vi "LuminosidadyTemperatura.vi"() -> ()   [LabVIEW 2021]
panel:
  out "Luz3":bool
  out "Luz2":bool
  in  "Sensor Presencia 3":bool
  in  "Sensor Presencia 2":bool
  in  "Sensor fotoelectrico":bool
  in  "Sensor Presencia 1":bool
  out "Calefactor":bool
  out "Ventilador":bool
  out "Indicador Analogico":dbl(knob) scale=0.0..45.0
  out "IndicadorTemp":dbl
  in  "Temperatura":dbl=15.0 min=15.0 max=26.0
  in  "ControlLuminosidad":dbl
  out "Luz1":bool
  out "Indicador 2":dbl
  out "Indicador":dbl
  out "Iluminacion 3":dbl(slide) scale=0.0..100.0
  out "Iluminacion 2":dbl(slide) scale=0.0..100.0
  out "Iluminacion 1":dbl(slide) scale=0.0..100.0
  out "Datos para DAQ 1":dbl
  in  "stop":bool
  # "Tablero de Monitoreo"
  # "Control de Luminosidad"
  # "Control de Temperatura"
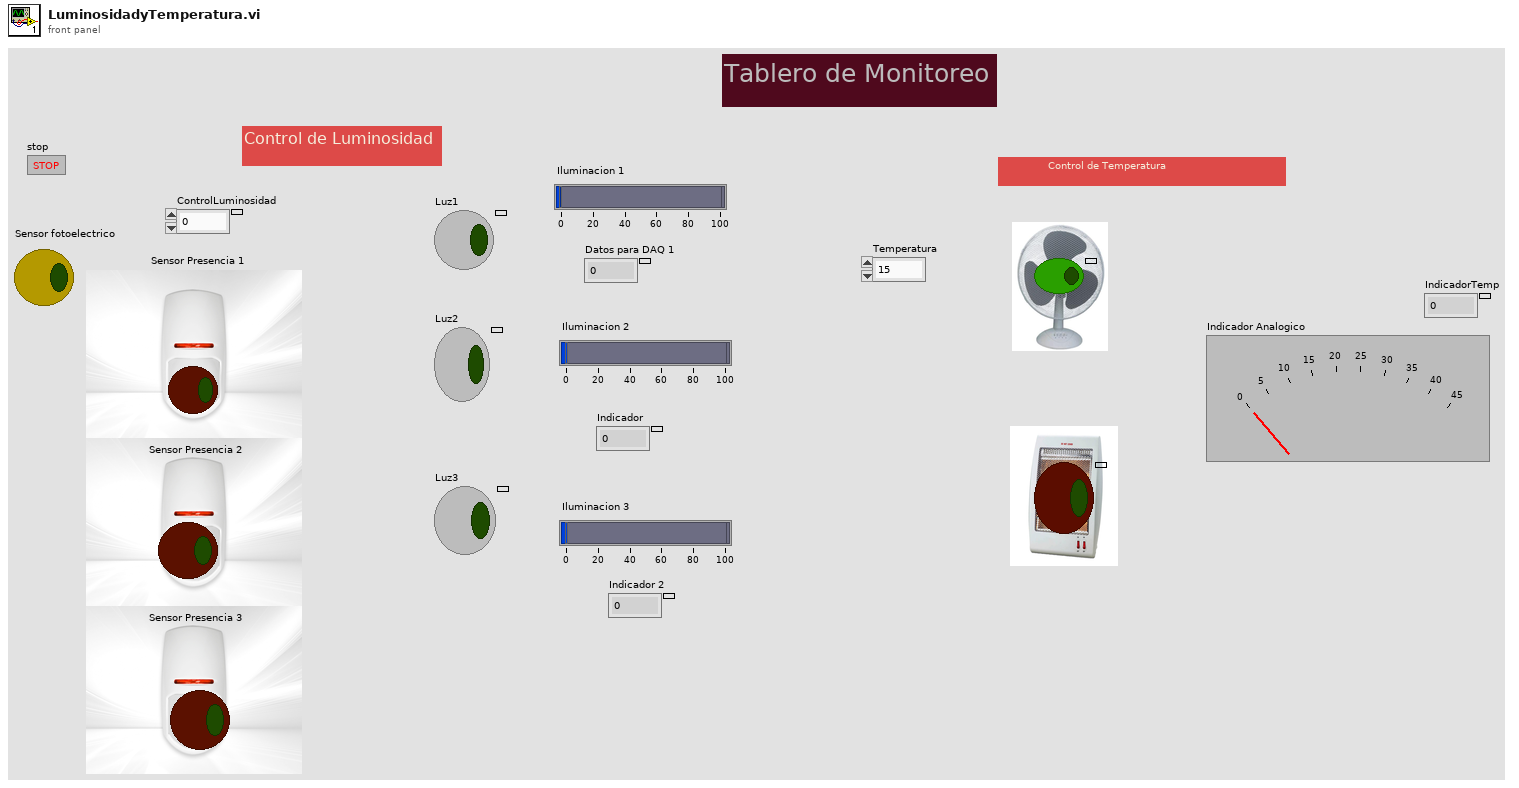
[diagram p1: front panel]
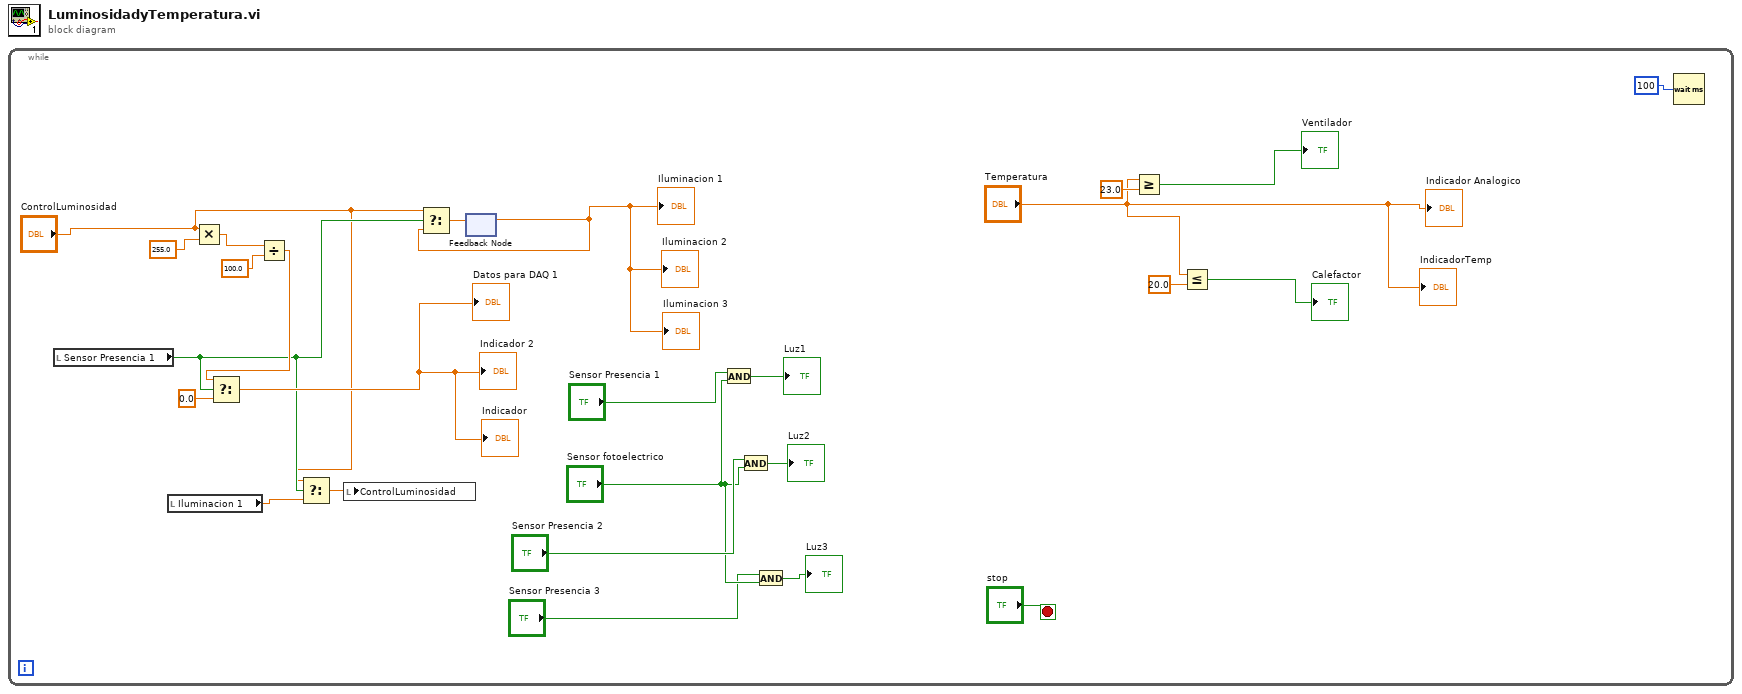
[diagram p0: block diagram]
diagram:
  n1 = while {
    stop <- "stop" stop-if-true
    n2 = local read "Sensor Presencia 1"() -> (w16:bool)
    n3 = local read "Iluminacion 1"() -> (w15:dbl)
    n4 = Multiply(x="ControlLuminosidad", y=255.0) -> (x*y=w23:dbl)
    n5 = Divide(x=w23, y=100.0) -> (x/y=w21:dbl)
    n6 = Select(t=w21, s=w16, f=0.0) -> (s? t:f=→"Datos para DAQ 1" →"Indicador 2" →"Indicador":dbl)
    n7 = Select(t="ControlLuminosidad", s=w16, f=w15) -> (s? t:f=w14:dbl)
    n8 = local write "ControlLuminosidad"(w14) -> ()
    n9 = feedback #1() -> (w18:dbl)  [unwired: 1 in]
    "Iluminacion 1" <- w18
    "Iluminacion 2" <- w18
    "Iluminacion 3" <- w18
    n10 = Select(t="ControlLuminosidad", s=w16, f=w18) -> (s? t:f=w19:dbl)
    n11 = feedback-in #1(w19) -> ()
    n12 = And(x="Sensor Presencia 1", y="Sensor fotoelectrico") -> (x .and. y?=→"Luz1":bool)
    n13 = And(x="Sensor Presencia 2", y="Sensor fotoelectrico") -> (x .and. y?=→"Luz2":bool)
    n14 = And(x="Sensor Presencia 3", y="Sensor fotoelectrico") -> (x .and. y?=→"Luz3":bool)
    n15 = Greater Or Equal?(x="Temperatura", y=23.0) -> (x >= y?=→"Ventilador":bool)
    n16 = Less Or Equal?(x="Temperatura", y=20.0) -> (x <= y?=→"Calefactor":bool)
    n17 = Wait (ms)(milliseconds to wait=u32 100) -> ()  [unwired: 1 out]
    "Indicador Analogico" <- "Temperatura"
    "IndicadorTemp" <- "Temperatura"
  }
